vi "loadplaylist.vi"(0 "Boolesch-ref":refnum<vi>, 1 "deutsch?":bool, 2 "input-array":string[](array[string]), 5 "ProgressBar-ref":refnum<k24>, 7 "playlist-input":string[](array[string]), 9 "pfade-in":string[](array[string]), 11 "symbole-in":dbl[](array[numeric]), 12 "ab position":dbl, 13 "ab position?":bool, 14 "von input-array?":bool) -> (4 "symbole-out":dbl[](array[numeric]), 8 "playlist-output":string[](array[string]), 15 "pfade-out":string[](array[string]))   [LabVIEW 2012]
uses:
  System.Windows.Forms
  <vilib>/Utility/error.llb/DialogType.ctl
  <vilib>/Utility/file.llb/Read From Spreadsheet File (string).vi
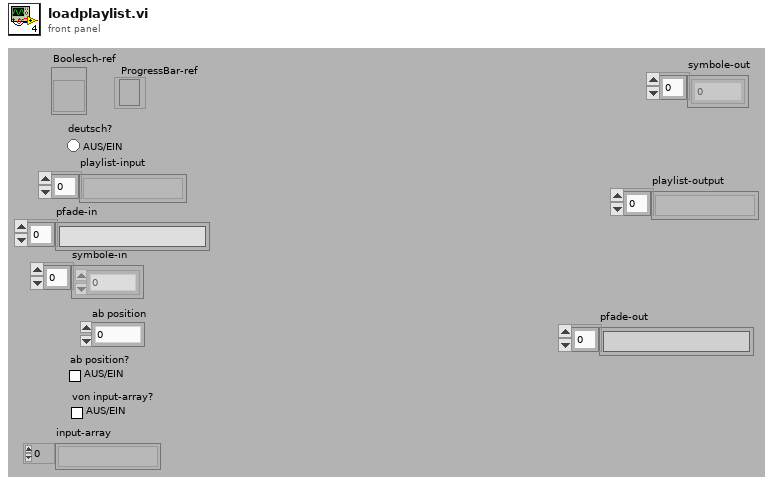
[diagram p1: front panel]
types:
  T1 = typedef "DialogType.ctl" = u16
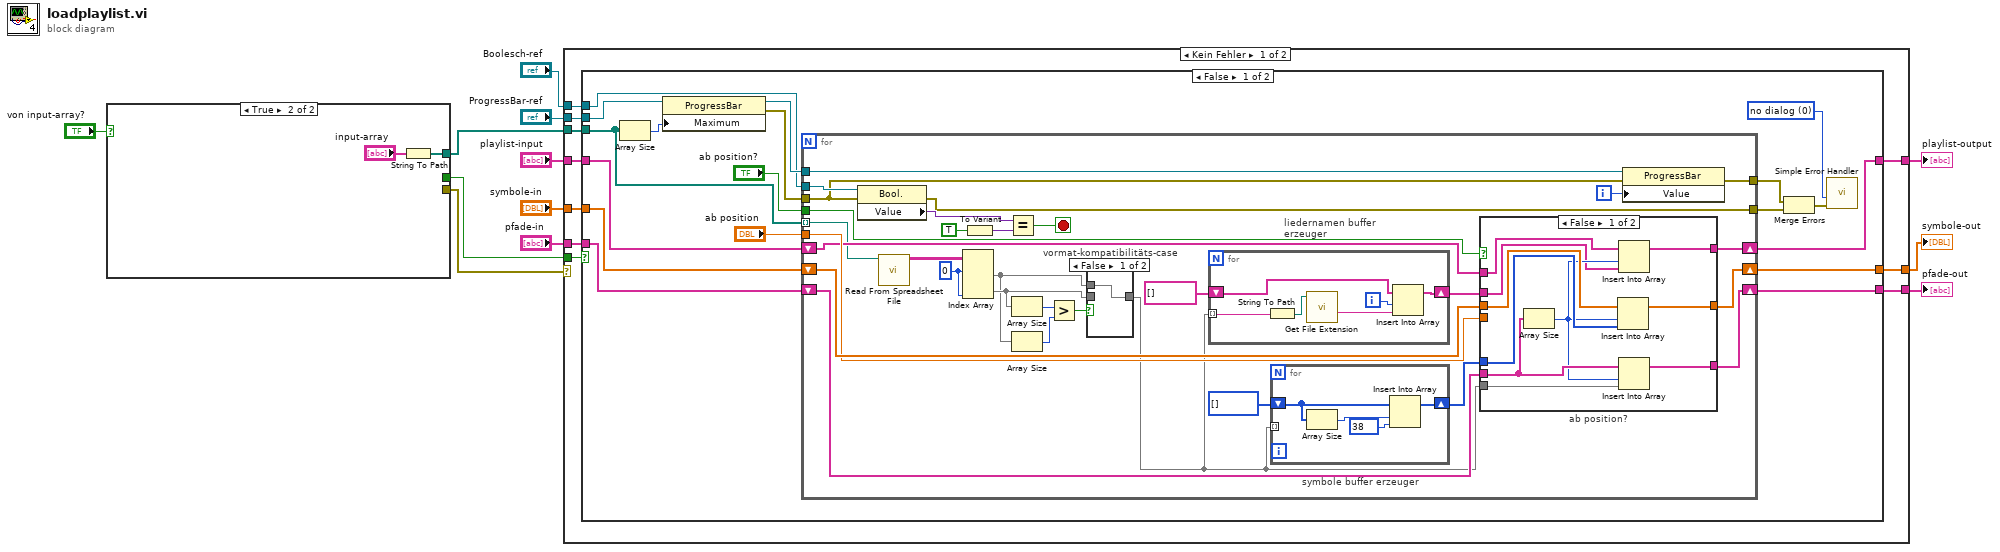
[diagram p0: block diagram]
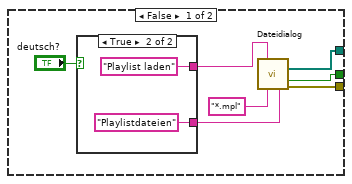
[diagram p2: hidden frame]
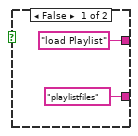
[diagram p3: hidden frame]
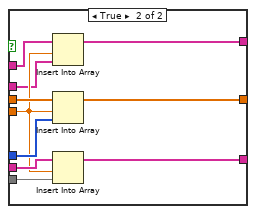
[diagram p5: hidden frame]
diagram:
  n1 = case shown="True" "von input-array?" {
    tunnel: [w15 _] -> w12
    tunnel: [w14 _] -> w11
    tunnel: [w13 w25] -> w10
    frame False {
      n2 = case shown="True" "deutsch?" {
        tunnel: ["load Playlist" ("Eingabeaufforderung") "Playlist laden" ("Eingabeaufforderung")] -> w18
        tunnel: ["playlistfiles" "Playlistdateien"] -> w17
        frame False {
        }
        frame True {
        }
      }
      n3 = call "Dateidialog"("prompt"=w18, "pattern (all files)"="*.mpl", "pattern label"=w17) -> ("selected paths"=w13:path[], "cancelled"=w15:bool, "error out"=w14:errorcluster)  [unwired: 4 in, 6 out]
    }
    frame True {
      n4 = String To Path(string="input-array") -> (path=w25:path[])
    }
  }
  n5 = case shown="Kein Fehler" w11 {
    tunnel: w12 -> [w35 _]
    tunnel: [w34 w122] -> w5
    tunnel: "pfade-in" -> [w33 w122]
    tunnel: w10 -> [w32 _]
    tunnel: "ProgressBar-ref" -> [w31 _]
    tunnel: "Boolesch-ref" -> [w30 _]
    tunnel: [w29 w121] -> w7
    tunnel: "symbole-in" -> [w28 w121]
    tunnel: "playlist-input" -> [w27 w120]
    tunnel: [w26 w120] -> w2
    frame No Error {
      n6 = case shown="False" w35 {
        tunnel: [w52 w119] -> w34
        tunnel: w33 -> [w53 w119]
        tunnel: w32 -> [w51 _]
        tunnel: w31 -> [w49 _]
        tunnel: w30 -> [w47 _]
        tunnel: [w45 w118] -> w29
        tunnel: w28 -> [w46 w118]
        tunnel: w27 -> [w42 w117]
        tunnel: [w41 w117] -> w26
        frame False {
          w39 = T1 0 items=["no dialog", "OK message", "continue or stop message", "OK message + warnings", "continue/stop + warnings"] ("type of dialog (OK msg:1)")
          n7 = Array Size(array=w51) -> (size(s)=w50:i32)
          n8 = property class="ProgressBar"(reference=w49, "Maximum"=w50) -> (reference out=w48:refnum<k24>, error out=w40:errorcluster)  [unwired: 1 in]
          n9 = for {
            tunnel: w51 -> [w62] mode=indexing
            shift-right: [w83] -> w52
            shift-left: w53 -> [w84]
            tunnel: w48 -> [w82]
            tunnel: w47 -> [w80]
            shift-right: [w76] -> w45
            shift-left: w46 -> [w78]
            tunnel: "ab position?" -> [w75]
            tunnel: "ab position" -> [w74]
            shift-right: [w71] -> w41
            shift-left: w42 -> [w72]
            tunnel: w40 -> [w65]
            tunnel: [w64] -> w38
            tunnel: [w63] -> w36
            i -> [w81]
            stop <- w66 stop-if-true
            w60 = 0 ("Index (Zeile)")
            n10 = property class="Bool."(reference=w80, error in=w65) -> (error out=w63:errorcluster, "Value"=w67:variant)  [unwired: 1 out]
            n11 = call-poly <vilib>:"Read From Spreadsheet File.vi"("file path (dialog if empty)"=w62) -> ("all rows"=w55:string[][])  [unwired: 3 in, 7 out]
            n12 = Index Array(array=w55, index (row) #1=w60, index (col) #2=w60) -> (element #1=w56:string[], element #2=w57:string[])  [unwired: 2 in]
            n13 = To Variant(anything=TRUE) -> (Variant=w68:variant)
            n14 = Equal?(x=w67, y=w68) -> (x = y?=w66:bool)
            n15 = Array Size(array=w57) -> (size(s)=w59:i32)
            n16 = Array Size(array=w56) -> (size(s)=w61:i32)
            n17 = Greater?(x=w59, y=w61) -> (0:w58:bool)
            n18 = case "vormat-kompatibilitäts-case" shown="False" w58 {
              tunnel: [w85 w86] -> w54
              tunnel: w57 -> [_ w86]
              tunnel: w56 -> [w85 _]
              frame False {
              }
              frame True {
              }
            }
            n19 = for "liedernamen buffer erzeuger" {
              tunnel: w54 -> [w92] mode=indexing
              shift-right: [w87] -> w70
              shift-left: string[] [] -> [w90]
              i -> [w89]
              n20 = String To Path(string=w92) -> (path=w91:path)
              n21 = call <vilib>:"Get File Extension.vi"("file"=w91) -> ("filename without extension"=w88:string)  [unwired: 7 in, 3 out]
              n22 = Insert Into Array(array=w90, index=w89, new element=w88) -> (w87:string[])
            }
            n23 = for "symbole buffer erzeuger" {
              shift-right: [w94] -> w77
              shift-left: i32[] [] -> [w95]
              tunnel: w54 -> [_] mode=indexing
              n24 = Array Size(array=w95) -> (size(s)=w96:i32)
              n25 = Insert Into Array(array=w95, index=w96, new element=38) -> (w94:i32[])
            }
            n26 = case "ab position?" shown="False" w75 {
              tunnel: w84 -> [w106 w116]
              tunnel: w54 -> [w105 w115]
              tunnel: [w104 w114] -> w83
              tunnel: w74 -> [_ w108]
              tunnel: w78 -> [w103 w113]
              tunnel: w77 -> [w102 w112]
              tunnel: [w101 w111] -> w76
              tunnel: w72 -> [w100 w110]
              tunnel: [w97 w109] -> w71
              tunnel: w70 -> [w98 w107]
              frame False {
                n27 = Array Size(array=w106) -> (size(s)=w99:i32)
                n28 = Insert Into Array(array=w103, index=w99, new element=w102) -> (w101:dbl[])
                n29 = Insert Into Array(array=w100, index=w99, new element=w98) -> (w97:string[])
                n30 = Insert Into Array(array=w106, index=w99, new element=w105) -> (w104:string[])
              }
              frame True {
                n31 = Insert Into Array(array=w110, index=w108, new element=w107) -> (w109:string[])
                n32 = Insert Into Array(array=w113, index=w108, new element=w112) -> (w111:dbl[])
                n33 = Insert Into Array(array=w116, index=w108, new element=w115) -> (w114:string[])
              }
            }
            n34 = property class="ProgressBar"(reference=w82, error in=w65, "Value"=w81) -> (error out=w64:errorcluster)  [unwired: 1 out]
          }
          n35 = Merge Errors(w38, w36) -> (w37:errorcluster)
          n36 = call <vilib>:"Simple Error Handler.vi"("type of dialog (OK msg:1)"=w39, "error in (no error)"=w37) -> ()  [unwired: 1 in, 7 out]
        }
        frame True {
        }
      }
    }
    frame Error {
    }
  }
  "playlist-output" <- w2
  "symbole-out" <- w7
  "pfade-out" <- w5
